vi "niRFUtil RFHS Channelizer GetNumFilterTaps.vi"(0 "fs":dbl=1.0, 5 "Channel Specification":T1={"fc"=0.0, "fs"=1.0, "passBW"=0.0, "stopBW"=0.0, "Rejection (dB)"=0.0, "Flags"=0, "Reserved"=0} {"Flags" items=["None"=0, "Force Fractional"=1, "Use Multistage"=2, "Use Pretrigger Data "=256, "Frequency Shift Only"=4]; "fs" format="%#_8p"; "fc" format="%#_6p"; "stopBW" format="%#_6p"; "passBW" format="%#_6p"}, 7 "Fractional":bool, 9 "upsample":i32=1, 11 "downsample":dbl=1.0) -> (4 "#Filter Taps":i32)   [LabVIEW 2015, in "niRFUtil.lvlib"]
uses:
  niRFUtil.lvlib
  Includes/niRFUtil RFHS Channelizer ChannelSpecificationBase.ctl
  Includes/niRFUtil RFHS Channelizer ChannelFlags.ctl
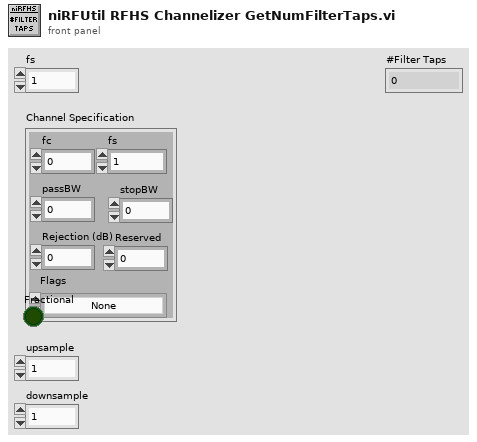
[diagram p1: front panel]
types:
  T1 = typedef "niRFUtil.lvlib/niRFUtil RFHS Channelizer ChannelSpecificationBase.ctl" = cluster{"fc":dbl, "fs":dbl, "passBW":dbl, "stopBW":dbl, "Rejection (dB)":dbl, "Flags":T2, "Reserved":i32}
  T2 = typedef "niRFUtil.lvlib/niRFUtil RFHS Channelizer ChannelFlags.ctl" = u32
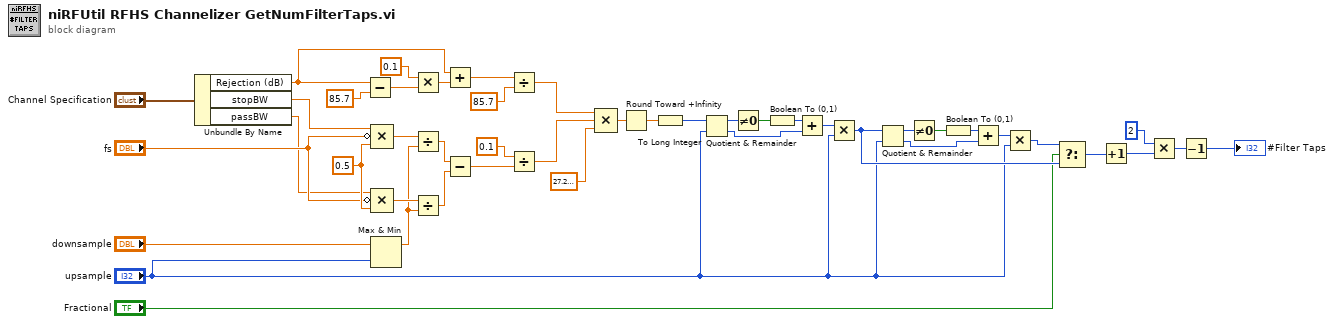
[diagram p0: block diagram]
diagram:
  w27 = 0.5 ("value")
  n1 = Unbundle By Name("Channel Specification") -> ("Rejection (dB)"=w34:dbl, "stopBW"=w6:dbl, "passBW"=w5:dbl)
  n2 = Subtract(x=w34, y=85.7) -> (x-y=w40:dbl)
  n3 = Compound Arithmetic op=MULTIPLY(w6, invert "fs", w27) -> (w36:dbl)
  n4 = Compound Arithmetic op=MULTIPLY(w5, invert "fs", w27) -> (w26:dbl)
  n5 = Max & Min(x="downsample", y="upsample") -> (max(x,y)=w23:dbl)  [unwired: 1 out]
  n6 = Multiply(x=0.1, y=w40) -> (x*y=w7:dbl)
  n7 = Divide(x=w36, y=w23) -> (x/y=w3:dbl)
  n8 = Divide(x=w26, y=w23) -> (x/y=w4:dbl)
  n9 = Add(x=w34, y=w7) -> (x+y=w38:dbl)
  n10 = Subtract(x=w3, y=w4) -> (x-y=w43:dbl)
  n11 = Divide(x=w38, y=85.7) -> (x/y=w2:dbl)
  n12 = Divide(x=0.1 ("y"), y=w43) -> (x/y=w37:dbl)
  n13 = Compound Arithmetic op=MULTIPLY(w2, w37, sgl 27.2 ("y")) -> (w35:dbl)
  n14 = Round Toward +Infinity(x=w35) -> (ceil(x): smallest int >= x=w28:dbl)
  n15 = To Long Integer(number=w28) -> (32bit integer=w16:i32)
  n16 = Quotient & Remainder(x=w16, y="upsample") -> (x-y*floor(x/y)=w33:i32, floor(x/y)=w30:i32)
  n17 = Not Equal To 0?(x=w33) -> (x != 0?=w32:bool)
  n18 = Boolean To (0,1)(Boolean=w32) -> (0, 1=w31:i16)
  n19 = Add(x=w31, y=w30) -> (x+y=w29:i32)
  n20 = Multiply(x=w29, y="upsample") -> (x*y=w17:i32)
  n21 = Quotient & Remainder(x=w17, y="upsample") -> (x-y*floor(x/y)=w19:i32, floor(x/y)=w1:i32)
  n22 = Not Equal To 0?(x=w19) -> (x != 0?=w20:bool)
  n23 = Boolean To (0,1)(Boolean=w20) -> (0, 1=w21:i16)
  n24 = Add(x=w21, y=w1) -> (x+y=w22:i32)
  n25 = Multiply(x=w22, y="upsample") -> (x*y=w18:i32)
  n26 = Select(t=w18, s="Fractional", f=w17) -> (s? t:f=w15:i32)
  n27 = Increment(x=w15) -> (x+1=w11:i32)
  n28 = Multiply(x=2, y=w11) -> (x*y=w9:i32)
  n29 = Decrement(x=w9) -> (x-1=→"#Filter Taps":i32)
